vi "Init.vi"(8 "error in (no error)":errorcluster, 11 "uService Template in":refnum<class "Dummy.lvclass">) -> (0 "error out":errorcluster, 3 "uService Template out":refnum<class "Dummy.lvclass">)   [LabVIEW 2020, in "Dummy.lvlib" / "Dummy.lvclass"]
uses:
  Dummy.lvclass
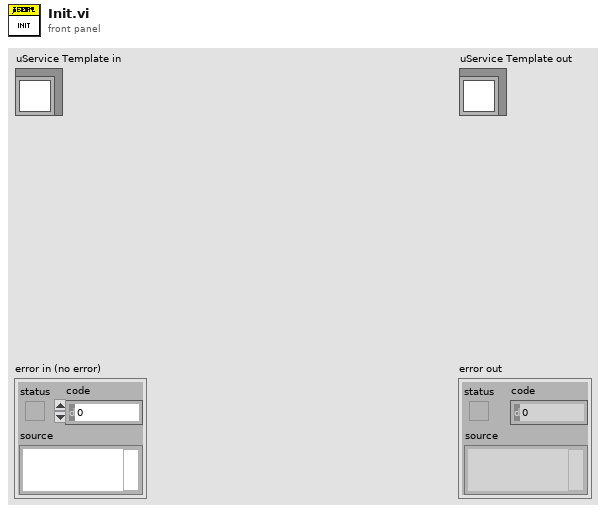
[diagram p1: front panel]
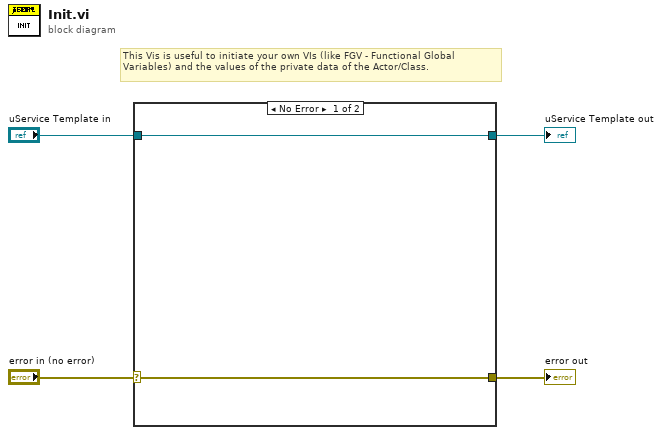
[diagram p0: block diagram]
diagram:
  # "This Vis is useful to initiate your own VIs (like FGV - Functional Global Variables) and the values of the private data of the Actor/Class."
  n1 = case shown="No Error" "error in (no error)" {
    selector: "error in (no error)" -> [w5 w7]
    tunnel: "uService Template in" -> [w6 w8]
    tunnel: [w6 w8] -> w4
    tunnel: [w5 w7] -> w3
    frame No Error {
    }
    frame Error {
    }
  }
  "error out" <- w3
  "uService Template out" <- w4
